vi "New.vi"(8 "error in (no error)":errorcluster, 9 "Goodbye Request":T1={"Error URI"="wamp.close.shut_down", "Message"="client disconnect"}, 10 "Serialisation":T2) -> (0 "error out":errorcluster, 3 "Goodbye JSON out":refnum<class "Goodbye.lvclass">)   [LabVIEW 2020, in "wamplv.lvlib" / "Goodbye.lvclass"]
uses:
  Goodbye.lvclass
  Goodbye.lvclass/Goodbye.ctl
  WAMP Client/API/TypeDefs/Serialisation.ctl
  WAMP Client/WAMP Client.lvclass
  WAMP Client/Private/TypeDef/GOODBYE Request Data.ctl
  wamplv.lvlib
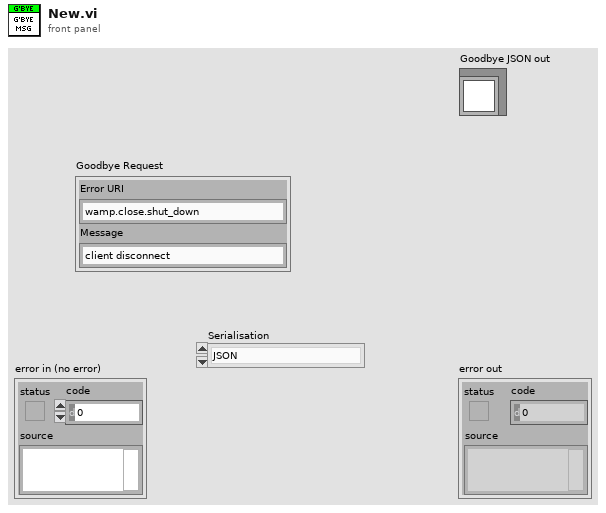
[diagram p1: front panel]
types:
  T1 = typedef "wamplv.lvlib/GOODBYE Request Data.ctl" = cluster{"Error URI":string, "Message":string}
  T2 = typedef "wamplv.lvlib/WAMP Client.lvclass/Serialisation.ctl" = enum16{"JSON", "MessagePack"}
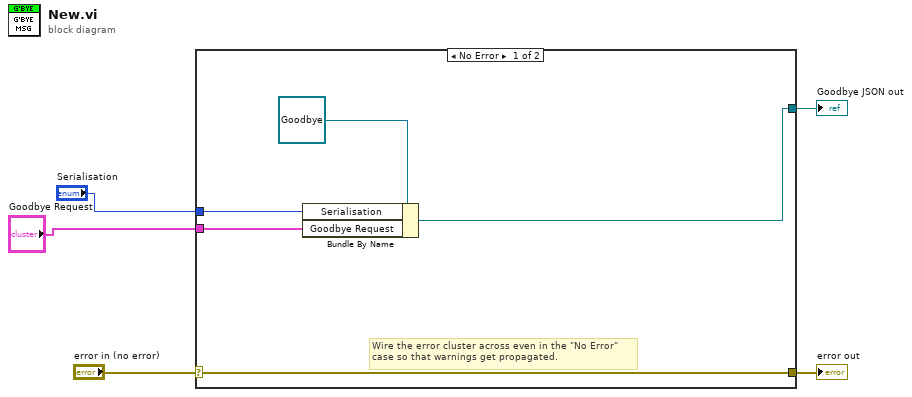
[diagram p0: block diagram]
diagram:
  n1 = case shown="No Error" "error in (no error)" {
    selector: "error in (no error)" -> [w10 w11]
    tunnel: [w10 w11] -> w4
    tunnel: [w7 _] -> w3
    tunnel: "Goodbye Request" -> [w9 _]
    tunnel: "Serialisation" -> [w8 _]
    frame No Error {
      # "Wire the error cluster across even in the \"No Error\"\ncase so that warnings get propagated."
      n2 = Bundle By Name(cluster=refnum<class "Goodbye.lvclass"> refnum ("wamplv.lvlib:Goodbye JSON.lvclass"), "Serialisation"=w8, "Goodbye Request"=w9) -> (w7:refnum<class "Goodbye.lvclass">)
    }
    frame Error {
    }
  }
  "error out" <- w4
  "Goodbye JSON out" <- w3
